vi "Get Object Properties.vi"(8 "error in (no error)":errorcluster, 11 "Item Ref in":T1 format="%.0x") -> (0 "error out":errorcluster, 1 "instance id":i32, 2 "class name":string, 3 "Item Ref out":T1 format="%.0x")   [LabVIEW 2019, in "HLA Custom Device System Explorer.lvlib"]
uses:
  HLA Custom Device System Explorer.lvlib
  <vilib>/NI VeriStand/Custom Device API/Custom Device Item Ref.ctl
  Shared/Constants.vi
  <vilib>/NI VeriStand/Custom Device API/Get Item Property (String).vi
  <vilib>/NI VeriStand/Custom Device API/Get Item Property (I32).vi
  Shared/HLA Custom Device Shared.lvlib
  <vilib>/NI VeriStand/Custom Device API/Custom Device API.lvlib
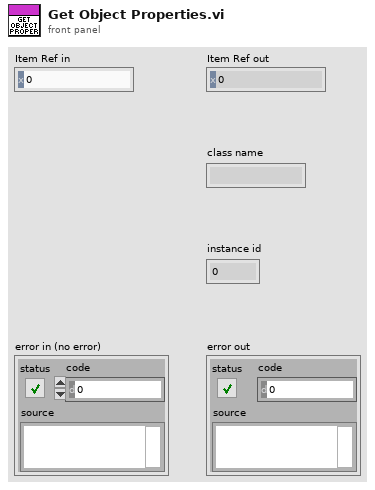
[diagram p1: front panel]
types:
  T1 = typedef "Custom Device API.lvlib/Custom Device Item Ref.ctl" = u64
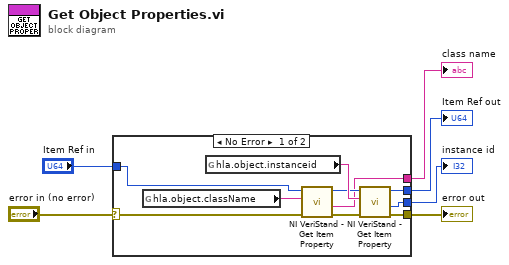
[diagram p0: block diagram]
diagram:
  n1 = case shown="No Error" "error in (no error)" {
    selector: "error in (no error)" -> [w9 w17]
    tunnel: [w12 w17] -> w6
    tunnel: "Item Ref in" -> [w11 w18]
    tunnel: [w10 w18] -> w4
    tunnel: [w8 _] -> w2
    tunnel: [w7 _] -> w1
    frame No Error {
      n2 = global read "Constants.vi" "hla.object.className"() -> (w14:string)
      n3 = global read "Constants.vi" "hla.object.instanceid"() -> (w16:string)
      n4 = call-poly <vilib>:"NI VeriStand - Get Item Property.vi"("error in (no error)"=w9, "Property Name"=w14, "Item Ref in"=w11) -> ("error out"=w15:errorcluster, "Value"=w7:string, "Item Ref out"=w13:T1)  [unwired: 5 in, 1 out]
      n5 = call-poly <vilib>:"NI VeriStand - Get Item Property.vi"("error in (no error)"=w15, "Property Name"=w16, "Item Ref in"=w13) -> ("error out"=w12:errorcluster, "Value"=w8:i32, "Item Ref out"=w10:T1)  [unwired: 5 in, 1 out]
    }
    frame Error {
    }
  }
  "error out" <- w6
  "Item Ref out" <- w4
  "instance id" <- w2
  "class name" <- w1
